vi "Auto Range(SR830).vi"(8 "error in (no error)":errorcluster, 11 "簇":T1={"initialize"=enum."SR830", "6221"={"6221 Resource"="GPIB0::24::INSTR", "Delta status"=FALSE, "电流|RMS(A)"=0.0}, "SR830+6221"={"source"=0, "Current(A)"=0.0, "阻抗(Ohm)"=0.0, "SR830 1"=FALSE, "SR830 2"=FALSE, "SR830 3"=FALSE, "SR830 4"=FALSE, "VISA 1"="", "VISA 2"="", "VISA 3"="", "VISA 4"="", "Reserve 1"=-1, "Reserve 2"=-1, "Reserve 3"=-1, "Reserve 4"=-1, "Sensitivity 1"=-1, "Sensitivity 2"=-1, "Sensitivity 3"=-1, "Sensitivity 4"=-1, "量程入 1"=0, "量程入 2"=0, "量程入 3"=0, "量程入 4"=0}, "2400"={"2400"=FALSE, "VISA"="GPIB0::9::INSTR", "Output Level (0)"=1e-05, "Compliance  Level (0.1)"=10.0}, "ch"={"ch"=[], "current"=[], "change?"=[], "holding current\nwhen change ch?"=FALSE}, "Instrument"={"325 Resource "="GPIB0::13::INSTR", "Input (0:A) 325"=0, "Heater Output (1:1) 325"=1, "340 Resource"="GPIB0::14::INSTR", "Input (0:A) 340"=0, "Loop (0: 1)"=0, "Input (0:B) 340"=1, "Loop (1: 1)"=0, "340 Status"=refnum, "Instrument Type"=enum."PPMS-Rotate", "quantum design"=refnum, "semaphore 325"=refnum, "TCP master instance"=refnum, "M24C Resource"="GPIB0::24::INSTR", "4G supply"="GPIB0::24::INSTR", "Temp Status 24C"=refnum, "Temp"=refnum, "9T信号"=refnum, "limit"={"Field limit"=0.0, "Field rate limit"=0.0, "Temp limit"=0.0, "Temp low limit"=0.0, "Temp rate limit "=0.0}, "4g supply status"=refnum, "vi路径"="", "in-plane"="", "out-plane"="", "in-plane signal"=FALSE, "out-plane signal"=FALSE, "in plane 信号"=refnum, "pzt volt"=refnum, "Aborting"=refnum, "数据文件"=refnum, "warning"=refnum, "750 visa"="", "750 rotate"="", "335 Status 2"=refnum, "335 Resource "="GPIB0::24::INSTR", "Input (0:A) 335"=0, "Input (0:B) 335"=1, "Heater Output (1:1) 335"=1, "semaphore 340"=refnum, "semaphore 335"=refnum, "325 Status"=refnum, "semaphore 750"=refnum, "750 field status"=refnum, "camg 振荡状态"=refnum, "列表框"=refnum, "编辑列表框？"=refnum, "camg Rate"=refnum, "行数"=refnum}, "2614B"={"2614B chA"=FALSE, "2614B chB"=FALSE, "VISA"=""}, "33522b"={"33522b resource name"="GPIB0::16::INSTR", "零电压"=0.0, "最大电压"=148.0, "间隔"=4.0, "最小电压"=-48.0, "PZT Scan?"=FALSE}, "gating type"=enum."2614(daul)", "层数"=0, "行数"=0, "是否处理"=[]} {"Instrument"."Loop (1: 1)" items=["1"=1, "2"=2]; "Instrument"."Loop (0: 1)" items=["1"=1, "2"=2]; "Instrument"."Input (0:B) 340" items=["A", "B", "C", "D"]; "Instrument"."Heater Output (1:1) 335" items=["1"=1, "2"=2]; "Instrument"."Input (0:B) 335" items=["A", "B"]; "Instrument"."Input (0:A) 335" items=["A", "B"]; "Instrument"."Heater Output (1:1) 325" items=["1"=1, "2"=2]; "Instrument"."Input (0:A) 325" items=["A", "B"]; "Instrument"."Input (0:A) 340" items=["1"=1, "2"=2]; "SR830+6221"."Sensitivity 4" items=["Auto Gain"=-1, "2 nV/fA"=0, "5 nV/fA"=1, "10 nV/fA"=2, "20 nV/fA"=3, "50 nV/fA"=4, "100 nV/fA"=5, "200 nV/fA"=6, "500 nV/fA"=7, "1 uV/pA"=8, "2 uV/pA"=9, "5 uV/pA"=10, "10 uV/pA"=11, "20 uV/pA"=12, "50 uV/pA"=13, "100 uV/pA"=14, "200 uV/pA"=15, "500 uV/pA"=16, "1 mV/nA"=17, "2 mV/nA"=18, "5 mV/nA"=19, "10 mV/nA"=20, "20 mV/nA"=21, "50 mV/nA"=22, "100 mV/nA"=23, "200 mV/nA"=24, "500 mV/mA"=25, "1 V/uA"=26]; "SR830+6221"."Sensitivity 3" items=["Auto Gain"=-1, "2 nV/fA"=0, "5 nV/fA"=1, "10 nV/fA"=2, "20 nV/fA"=3, "50 nV/fA"=4, "100 nV/fA"=5, "200 nV/fA"=6, "500 nV/fA"=7, "1 uV/pA"=8, "2 uV/pA"=9, "5 uV/pA"=10, "10 uV/pA"=11, "20 uV/pA"=12, "50 uV/pA"=13, "100 uV/pA"=14, "200 uV/pA"=15, "500 uV/pA"=16, "1 mV/nA"=17, "2 mV/nA"=18, "5 mV/nA"=19, "10 mV/nA"=20, "20 mV/nA"=21, "50 mV/nA"=22, "100 mV/nA"=23, "200 mV/nA"=24, "500 mV/mA"=25, "1 V/uA"=26]; "SR830+6221"."Sensitivity 1" items=["Auto Gain"=-1, "2 nV/fA"=0, "5 nV/fA"=1, "10 nV/fA"=2, "20 nV/fA"=3, "50 nV/fA"=4, "100 nV/fA"=5, "200 nV/fA"=6, "500 nV/fA"=7, "1 uV/pA"=8, "2 uV/pA"=9, "5 uV/pA"=10, "10 uV/pA"=11, "20 uV/pA"=12, "50 uV/pA"=13, "100 uV/pA"=14, "200 uV/pA"=15, "500 uV/pA"=16, "1 mV/nA"=17, "2 mV/nA"=18, "5 mV/nA"=19, "10 mV/nA"=20, "20 mV/nA"=21, "50 mV/nA"=22, "100 mV/nA"=23, "200 mV/nA"=24, "500 mV/mA"=25, "1 V/uA"=26]; "SR830+6221"."Sensitivity 2" items=["Auto Gain"=-1, "2 nV/fA"=0, "5 nV/fA"=1, "10 nV/fA"=2, "20 nV/fA"=3, "50 nV/fA"=4, "100 nV/fA"=5, "200 nV/fA"=6, "500 nV/fA"=7, "1 uV/pA"=8, "2 uV/pA"=9, "5 uV/pA"=10, "10 uV/pA"=11, "20 uV/pA"=12, "50 uV/pA"=13, "100 uV/pA"=14, "200 uV/pA"=15, "500 uV/pA"=16, "1 mV/nA"=17, "2 mV/nA"=18, "5 mV/nA"=19, "10 mV/nA"=20, "20 mV/nA"=21, "50 mV/nA"=22, "100 mV/nA"=23, "200 mV/nA"=24, "500 mV/mA"=25, "1 V/uA"=26]; "SR830+6221"."Reserve 4" items=["Auto Reserve"=-1, "High Reserve"=0, "Normal"=1, "Low Noise"=2]; "SR830+6221"."Reserve 3" items=["Auto Reserve"=-1, "High Reserve"=0, "Normal"=1, "Low Noise"=2]; "SR830+6221"."Reserve 2" items=["Auto Reserve"=-1, "High Reserve"=0, "Normal"=1, "Low Noise"=2]; "SR830+6221"."Reserve 1" items=["Auto Reserve"=-1, "High Reserve"=0, "Normal"=1, "Low Noise"=2]; "SR830+6221"."source" items=["SR830 1", "SR830 2", "SR830 3", "SR830 4"]}) -> (0 "错误输出":errorcluster)   [LabVIEW 2019, in "User lib.lvlib"]
uses:
  ctl/config.ctl
  <vilib>/NI/Modbus Library/API/Master/Modbus Master.lvclass
  ctl/initialize.ctl
  ctl/Instrument.ctl
  ctl/335 state.ctl
  ctl/Instrument Type.ctl
  lib/QDInstrument.dll
  ctl/limit.ctl
  ctl/9T mag field stauts.ctl
  ctl/warning.ctl
  ctl/Gating type.ctl
  User lib.lvlib
  lib/Stanford Research 830/Stanford Research 830.lvlib
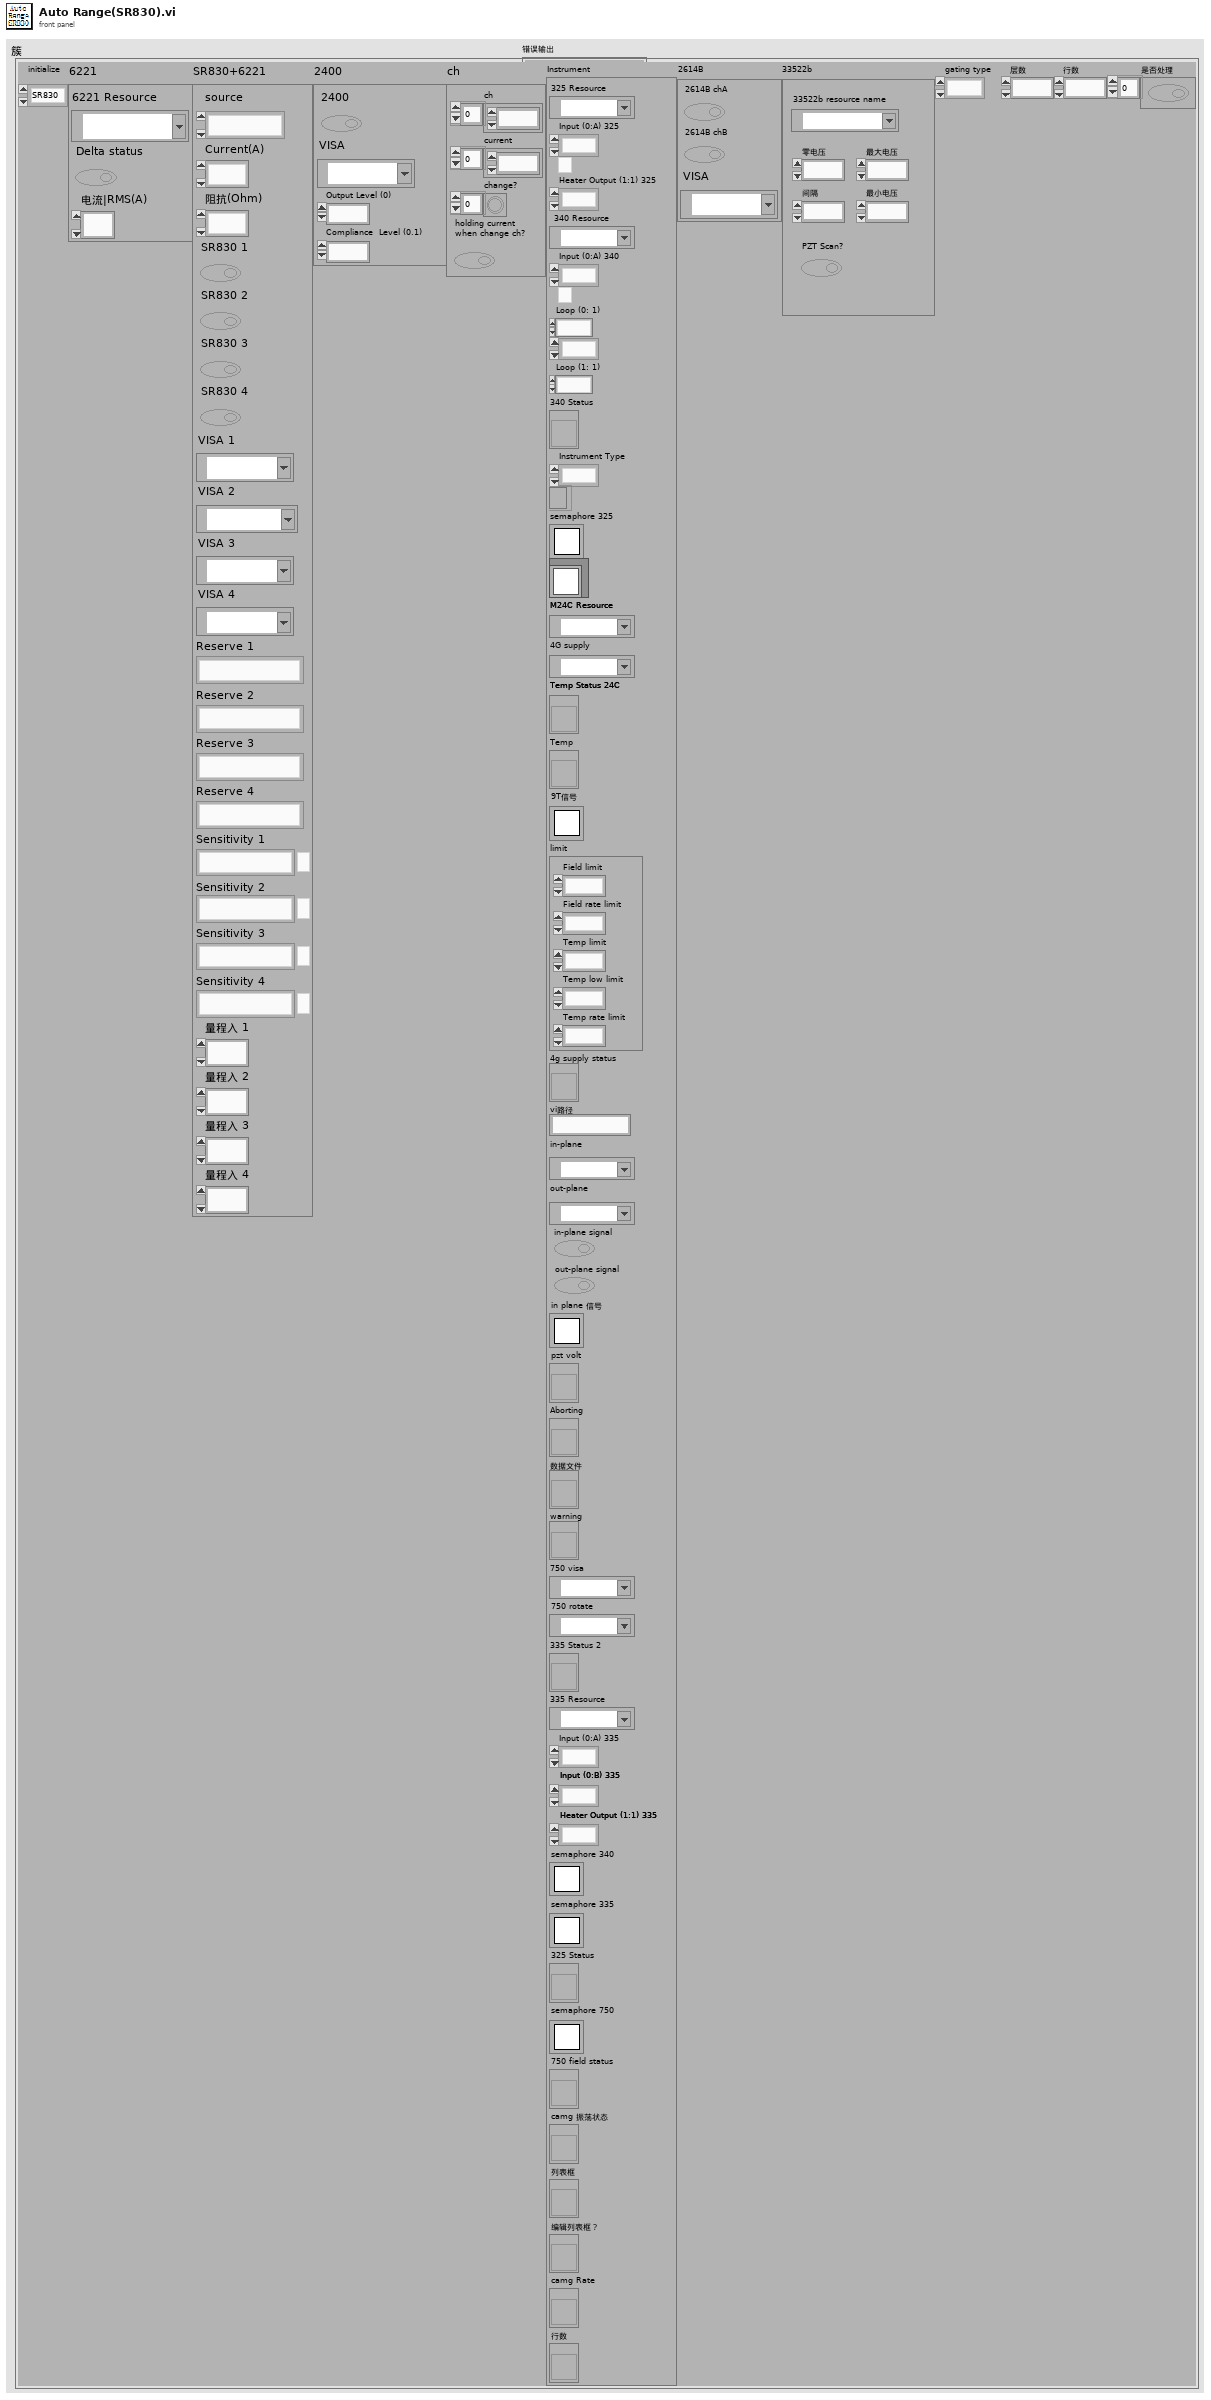
[diagram p1: front panel]
types:
  T1 = typedef "config.ctl" = cluster{"initialize":T2, "6221":cluster{"6221 Resource":refnum<visa-resource-name>, "Delta status":bool, "电流|RMS(A)":dbl}, "SR830+6221":cluster{"source":u16, "Current(A)":dbl, "阻抗(Ohm)":dbl, "SR830 1":bool, "SR830 2":bool, "SR830 3":bool, "SR830 4":bool, "VISA 1":refnum<visa-resource-name>, "VISA 2":refnum<visa-resource-name>, "VISA 3":refnum<visa-resource-name>, "VISA 4":refnum<visa-resource-name>, "Reserve 1":i16, "Reserve 2":i16, "Reserve 3":i16, "Reserve 4":i16, "Sensitivity 1":i16, "Sensitivity 2":i16, "Sensitivity 3":i16, "Sensitivity 4":i16, "量程入 1":i32, "量程入 2":i32, "量程入 3":i32, "量程入 4":i32}, "2400":cluster{"2400":bool, "VISA":refnum<visa-resource-name>, "Output Level (0)":dbl, "Compliance  Level (0.1)":dbl}, "ch":cluster{"ch":i32[], "current":dbl[], "change?":bool[], "holding current\nwhen change ch?":bool}, "Instrument":T3, "2614B":cluster{"2614B chA":bool, "2614B chB":bool, "VISA":refnum<visa-resource-name>}, "33522b":cluster{"33522b resource name":refnum<visa-resource-name>, "零电压":dbl, "最大电压":dbl, "间隔":dbl, "最小电压":dbl, "PZT Scan?":bool}, "gating type":T7, "层数":i32, "行数":i32, "是否处理":bool[]}
  T2 = typedef "initialize.ctl" = enum16{"SR830", "keithley6221-SR830", "Delta", "Delta-tunnelling", "keithley6221-2182-DC", "PZT", "4200"}
  T3 = typedef "Instrument.ctl" = cluster{"325 Resource ":refnum<visa-resource-name>, "Input (0:A) 325":u16, "Heater Output (1:1) 325":u16, "340 Resource":refnum<visa-resource-name>, "Input (0:A) 340":u16, "Loop (0: 1)":u16, "Input (0:B) 340":u16, "Loop (1: 1)":u16, "340 Status":refnum<vi>, "Instrument Type":T4, "quantum design":refnum<k24>, "semaphore 325":T5, "TCP master instance":refnum<class "Modbus Master.lvclass">, "M24C Resource":refnum<visa-resource-name>, "4G supply":refnum<visa-resource-name>, "Temp Status 24C":refnum<vi>, "Temp":refnum<vi>, "9T信号":T5, "limit":T6, "4g supply status":refnum<vi>, "vi路径":string, "in-plane":refnum<visa-resource-name>, "out-plane":refnum<visa-resource-name>, "in-plane signal":bool, "out-plane signal":bool, "in plane 信号":T5, "pzt volt":refnum<vi>, "Aborting":refnum<vi>, "数据文件":refnum<vi>, "warning":refnum<vi>, "750 visa":refnum<visa-resource-name>, "750 rotate":refnum<visa-resource-name>, "335 Status 2":refnum<vi>, "335 Resource ":refnum<visa-resource-name>, "Input (0:A) 335":u16, "Input (0:B) 335":u16, "Heater Output (1:1) 335":u16, "semaphore 340":T5, "semaphore 335":T5, "325 Status":refnum<vi>, "semaphore 750":T5, "750 field status":refnum<vi>, "camg 振荡状态":refnum<vi>, "列表框":refnum<vi>, "编辑列表框？":refnum<vi>, "camg Rate":refnum<vi>, "行数":refnum<vi>}
  T4 = typedef "Instrument Type.ctl" = enum16{"PPMS", "VersaLab", "DynaCool", "SVSM", "PPMS-Rotate", "Lakeshore335", "lengtou2", "9T mag", "9T cmag rotate", "test"}
  T5 = typedef "Semaphore RefNum" = refnum<k1>
  T6 = typedef "limit.ctl" = cluster{"Field limit":dbl, "Field rate limit":dbl, "Temp limit":dbl, "Temp low limit":dbl, "Temp rate limit ":dbl}
  T7 = typedef "Gating type.ctl" = enum32{"null", "2614(daul)", "2400", "6517B"}
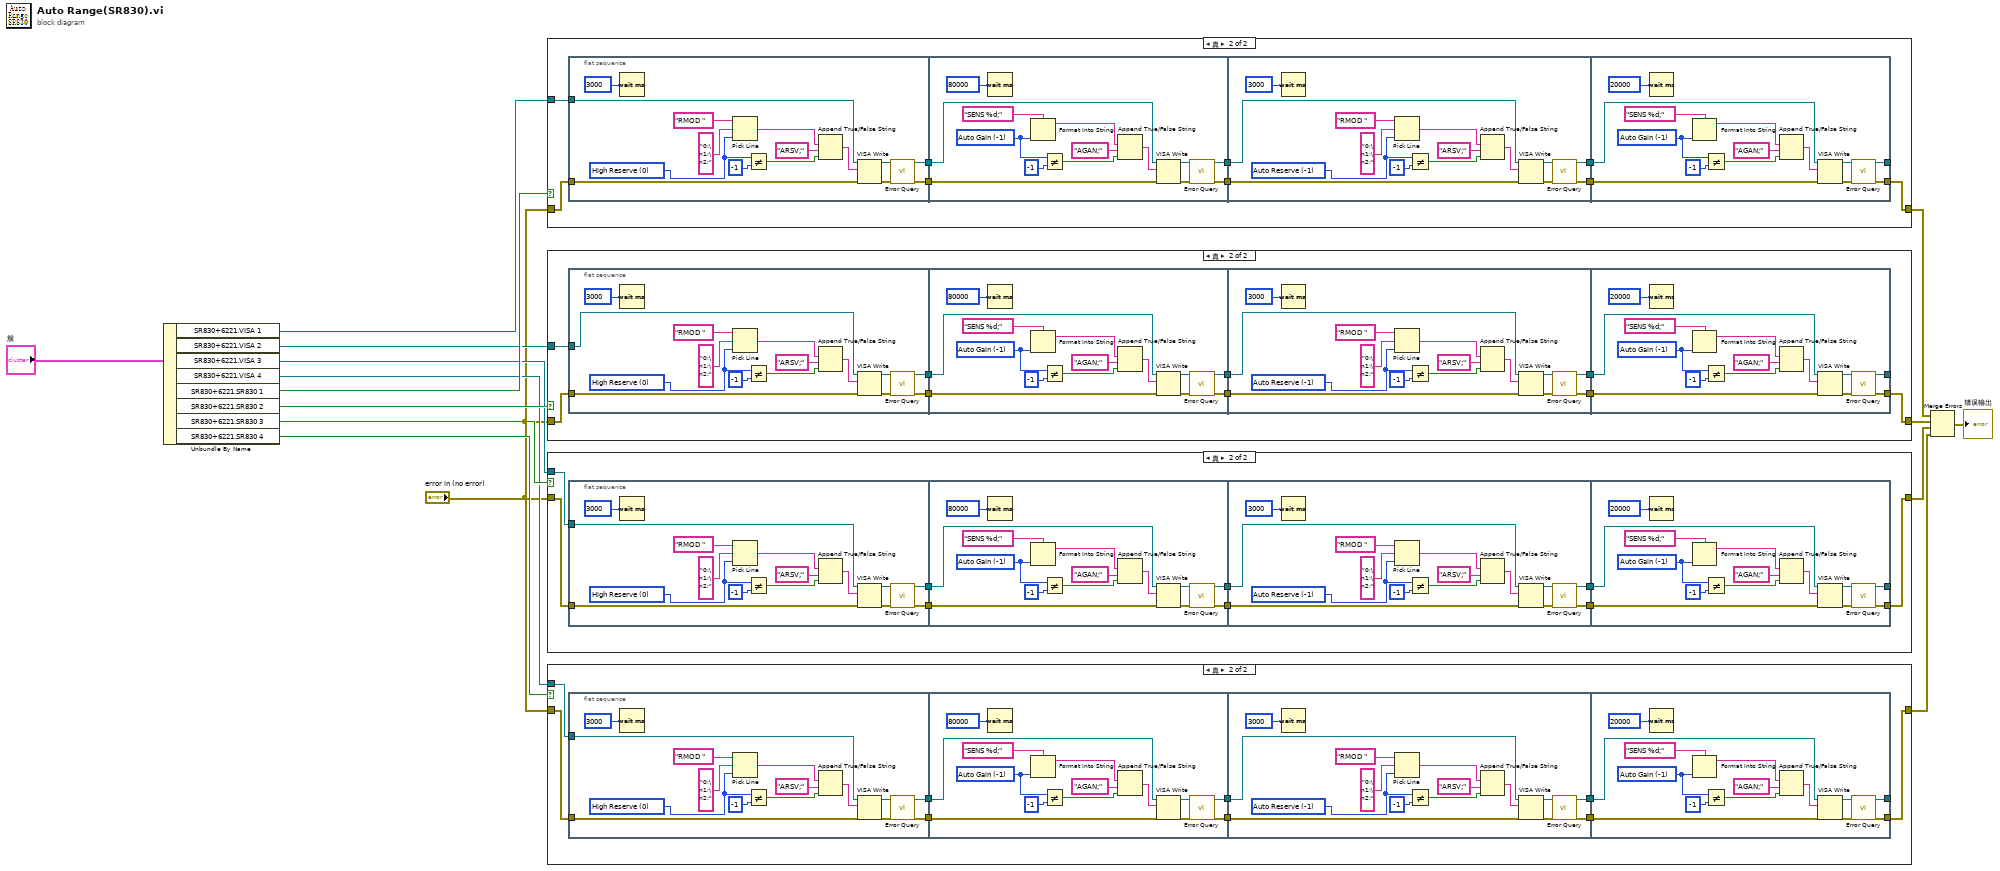
[diagram p0: block diagram]
diagram:
  n1 = Unbundle By Name("簇") -> ("SR830+6221.VISA 1"=w9:refnum<visa-resource-name>, "SR830+6221.VISA 2"=w7:refnum<visa-resource-name>, "SR830+6221.VISA 3"=w5:refnum<visa-resource-name>, "SR830+6221.VISA 4"=w3:refnum<visa-resource-name>, "SR830+6221.SR830 1"=w13:bool, "SR830+6221.SR830 2"=w12:bool, "SR830+6221.SR830 3"=w11:bool, "SR830+6221.SR830 4"=w10:bool)
  n2 = case shown="真" w13 {
    tunnel: w9 -> [_ w19]
    tunnel: "error in (no error)" -> [w16 w18]
    tunnel: [w16 w17] -> w8
    frame False {
    }
    frame True {
      n3 = flat-sequence {
        tunnel: w19 -> [w31]
        tunnel: w18 -> [w30]
        tunnel: [w27] -> w25
        tunnel: [w28] -> w24
        tunnel: [w43] -> w23
        tunnel: [w42] -> w22
        tunnel: w25 -> [w45]
        tunnel: w24 -> [w44]
        tunnel: w23 -> [w60]
        tunnel: w22 -> [w61]
        tunnel: [w57] -> w20
        tunnel: [w56] -> w21
        tunnel: w21 -> [w73]
        tunnel: w20 -> [w74]
        tunnel: [w71] -> w17
        tunnel: [w70] -> _
        frame #0 {
          w38 = i16 0 items=["Auto Reserve"=-1, "High Reserve"=0, "Normal"=1, "Low Noise"=2] ("Dynamic Reserve (-1: Auto Reserve)")
          n4 = Wait (ms)(milliseconds to wait=u32 3000 ("等待时间（毫秒）")) -> ()  [unwired: 1 out]
          n5 = Pick Line(string ("")="RMOD ", multi-line string="0;\n1;\n2;", line index=w38) -> (output string=w40:string)
          n6 = Not Equal?(x=w38, y=i16 -1) -> (x != y?=w39:bool)
          n7 = Append True/False String(1:w39, 2:"ARSV;" ("false string"), 3:w40) -> (0:w29:string)  [unwired: 1 in]
          n8 = VISA Write(VISA resource name=w31, write buffer=w29, error in (no error)=w30) -> (VISA resource name out=w32:refnum<visa-resource-name>, error out=w33:errorcluster)  [unwired: 1 out]
          n9 = call "Error Query.vi"("error in (no error)"=w33, "VISA resource name"=w32) -> ("error out"=w27:errorcluster, "VISA resource name out"=w28:refnum<visa-resource-name>)  [unwired: 7 in, 1 out]
        }
        frame #1 {
          w48 = i16 -1 items=["Auto Gain"=-1, "2 nV/fA"=0, "5 nV/fA"=1, "10 nV/fA"=2, "20 nV/fA"=3, "50 nV/fA"=4, "100 nV/fA"=5, "200 nV/fA"=6, "500 nV/fA"=7, "1 uV/pA"=8, "2 uV/pA"=9, "5 uV/pA"=10, "10 uV/pA"=11, "20 uV/pA"=12, "50 uV/pA"=13, "100 uV/pA"=14, "200 uV/pA"=15, "500 uV/pA"=16, "1 mV/nA"=17, "2 mV/nA"=18, "5 mV/nA"=19, "10 mV/nA"=20, "20 mV/nA"=21, "50 mV/nA"=22, "100 mV/nA"=23, "200 mV/nA"=24, "500 mV/mA"=25, "1 V/uA"=26] ("Sensitivity (-1: Auto gain)")
          n10 = Wait (ms)(milliseconds to wait=u32 80000 ("等待时间（毫秒）")) -> ()  [unwired: 1 out]
          n11 = Format Into String(format string="SENS %d;", w48) -> (resulting string=w51:string)  [unwired: 2 in, 1 out]
          n12 = Not Equal?(x=w48, y=i16 -1) -> (x != y?=w50:bool)
          n13 = Append True/False String(1:w50, 2:"AGAN;" ("false string"), 3:w51) -> (0:w54:string)  [unwired: 1 in]
          n14 = VISA Write(VISA resource name=w44, write buffer=w54, error in (no error)=w45) -> (VISA resource name out=w52:refnum<visa-resource-name>, error out=w53:errorcluster)  [unwired: 1 out]
          n15 = call "Error Query.vi"("error in (no error)"=w53, "VISA resource name"=w52) -> ("error out"=w43:errorcluster, "VISA resource name out"=w42:refnum<visa-resource-name>)  [unwired: 7 in, 1 out]
        }
        frame #2 {
          w67 = i16 -1 items=["Auto Reserve"=-1, "High Reserve"=0, "Normal"=1, "Low Noise"=2] ("Dynamic Reserve (-1: Auto Reserve)")
          n16 = Wait (ms)(milliseconds to wait=u32 3000 ("等待时间（毫秒）")) -> ()  [unwired: 1 out]
          n17 = Pick Line(string ("")="RMOD ", multi-line string="0;\n1;\n2;", line index=w67) -> (output string=w69:string)
          n18 = Not Equal?(x=w67, y=i16 -1) -> (x != y?=w68:bool)
          n19 = Append True/False String(1:w68, 2:"ARSV;" ("false string"), 3:w69) -> (0:w62:string)  [unwired: 1 in]
          n20 = VISA Write(VISA resource name=w61, write buffer=w62, error in (no error)=w60) -> (VISA resource name out=w58:refnum<visa-resource-name>, error out=w59:errorcluster)  [unwired: 1 out]
          n21 = call "Error Query.vi"("error in (no error)"=w59, "VISA resource name"=w58) -> ("error out"=w56:errorcluster, "VISA resource name out"=w57:refnum<visa-resource-name>)  [unwired: 7 in, 1 out]
        }
        frame #3 {
          w77 = i16 -1 items=["Auto Gain"=-1, "2 nV/fA"=0, "5 nV/fA"=1, "10 nV/fA"=2, "20 nV/fA"=3, "50 nV/fA"=4, "100 nV/fA"=5, "200 nV/fA"=6, "500 nV/fA"=7, "1 uV/pA"=8, "2 uV/pA"=9, "5 uV/pA"=10, "10 uV/pA"=11, "20 uV/pA"=12, "50 uV/pA"=13, "100 uV/pA"=14, "200 uV/pA"=15, "500 uV/pA"=16, "1 mV/nA"=17, "2 mV/nA"=18, "5 mV/nA"=19, "10 mV/nA"=20, "20 mV/nA"=21, "50 mV/nA"=22, "100 mV/nA"=23, "200 mV/nA"=24, "500 mV/mA"=25, "1 V/uA"=26] ("Sensitivity (-1: Auto gain)")
          n22 = Wait (ms)(milliseconds to wait=u32 20000 ("等待时间（毫秒）")) -> ()  [unwired: 1 out]
          n23 = Format Into String(format string="SENS %d;", w77) -> (resulting string=w80:string)  [unwired: 2 in, 1 out]
          n24 = Not Equal?(x=w77, y=i16 -1) -> (x != y?=w79:bool)
          n25 = Append True/False String(1:w79, 2:"AGAN;" ("false string"), 3:w80) -> (0:w83:string)  [unwired: 1 in]
          n26 = VISA Write(VISA resource name=w74, write buffer=w83, error in (no error)=w73) -> (VISA resource name out=w81:refnum<visa-resource-name>, error out=w82:errorcluster)  [unwired: 1 out]
          n27 = call "Error Query.vi"("error in (no error)"=w82, "VISA resource name"=w81) -> ("error out"=w71:errorcluster, "VISA resource name out"=w70:refnum<visa-resource-name>)  [unwired: 7 in, 1 out]
        }
      }
    }
  }
  n28 = case shown="真" w12 {
    tunnel: w7 -> [_ w87]
    tunnel: "error in (no error)" -> [w84 w86]
    tunnel: [w84 w85] -> w6
    frame False {
    }
    frame True {
      n29 = flat-sequence {
        tunnel: w87 -> [w99]
        tunnel: w86 -> [w98]
        tunnel: [w95] -> w93
        tunnel: [w96] -> w92
        tunnel: [w111] -> w91
        tunnel: [w110] -> w90
        tunnel: w93 -> [w113]
        tunnel: w92 -> [w112]
        tunnel: w91 -> [w128]
        tunnel: w90 -> [w129]
        tunnel: [w125] -> w88
        tunnel: [w124] -> w89
        tunnel: w89 -> [w141]
        tunnel: w88 -> [w142]
        tunnel: [w139] -> w85
        tunnel: [w138] -> _
        frame #0 {
          w106 = i16 0 items=["Auto Reserve"=-1, "High Reserve"=0, "Normal"=1, "Low Noise"=2] ("Dynamic Reserve (-1: Auto Reserve)")
          n30 = Wait (ms)(milliseconds to wait=u32 3000 ("等待时间（毫秒）")) -> ()  [unwired: 1 out]
          n31 = Pick Line(string ("")="RMOD ", multi-line string="0;\n1;\n2;", line index=w106) -> (output string=w108:string)
          n32 = Not Equal?(x=w106, y=i16 -1) -> (x != y?=w107:bool)
          n33 = Append True/False String(1:w107, 2:"ARSV;" ("false string"), 3:w108) -> (0:w97:string)  [unwired: 1 in]
          n34 = VISA Write(VISA resource name=w99, write buffer=w97, error in (no error)=w98) -> (VISA resource name out=w100:refnum<visa-resource-name>, error out=w101:errorcluster)  [unwired: 1 out]
          n35 = call "Error Query.vi"("error in (no error)"=w101, "VISA resource name"=w100) -> ("error out"=w95:errorcluster, "VISA resource name out"=w96:refnum<visa-resource-name>)  [unwired: 7 in, 1 out]
        }
        frame #1 {
          w116 = i16 -1 items=["Auto Gain"=-1, "2 nV/fA"=0, "5 nV/fA"=1, "10 nV/fA"=2, "20 nV/fA"=3, "50 nV/fA"=4, "100 nV/fA"=5, "200 nV/fA"=6, "500 nV/fA"=7, "1 uV/pA"=8, "2 uV/pA"=9, "5 uV/pA"=10, "10 uV/pA"=11, "20 uV/pA"=12, "50 uV/pA"=13, "100 uV/pA"=14, "200 uV/pA"=15, "500 uV/pA"=16, "1 mV/nA"=17, "2 mV/nA"=18, "5 mV/nA"=19, "10 mV/nA"=20, "20 mV/nA"=21, "50 mV/nA"=22, "100 mV/nA"=23, "200 mV/nA"=24, "500 mV/mA"=25, "1 V/uA"=26] ("Sensitivity (-1: Auto gain)")
          n36 = Wait (ms)(milliseconds to wait=u32 80000 ("等待时间（毫秒）")) -> ()  [unwired: 1 out]
          n37 = Format Into String(format string="SENS %d;", w116) -> (resulting string=w119:string)  [unwired: 2 in, 1 out]
          n38 = Not Equal?(x=w116, y=i16 -1) -> (x != y?=w118:bool)
          n39 = Append True/False String(1:w118, 2:"AGAN;" ("false string"), 3:w119) -> (0:w122:string)  [unwired: 1 in]
          n40 = VISA Write(VISA resource name=w112, write buffer=w122, error in (no error)=w113) -> (VISA resource name out=w120:refnum<visa-resource-name>, error out=w121:errorcluster)  [unwired: 1 out]
          n41 = call "Error Query.vi"("error in (no error)"=w121, "VISA resource name"=w120) -> ("error out"=w111:errorcluster, "VISA resource name out"=w110:refnum<visa-resource-name>)  [unwired: 7 in, 1 out]
        }
        frame #2 {
          w135 = i16 -1 items=["Auto Reserve"=-1, "High Reserve"=0, "Normal"=1, "Low Noise"=2] ("Dynamic Reserve (-1: Auto Reserve)")
          n42 = Wait (ms)(milliseconds to wait=u32 3000 ("等待时间（毫秒）")) -> ()  [unwired: 1 out]
          n43 = Pick Line(string ("")="RMOD ", multi-line string="0;\n1;\n2;", line index=w135) -> (output string=w137:string)
          n44 = Not Equal?(x=w135, y=i16 -1) -> (x != y?=w136:bool)
          n45 = Append True/False String(1:w136, 2:"ARSV;" ("false string"), 3:w137) -> (0:w130:string)  [unwired: 1 in]
          n46 = VISA Write(VISA resource name=w129, write buffer=w130, error in (no error)=w128) -> (VISA resource name out=w126:refnum<visa-resource-name>, error out=w127:errorcluster)  [unwired: 1 out]
          n47 = call "Error Query.vi"("error in (no error)"=w127, "VISA resource name"=w126) -> ("error out"=w124:errorcluster, "VISA resource name out"=w125:refnum<visa-resource-name>)  [unwired: 7 in, 1 out]
        }
        frame #3 {
          w145 = i16 -1 items=["Auto Gain"=-1, "2 nV/fA"=0, "5 nV/fA"=1, "10 nV/fA"=2, "20 nV/fA"=3, "50 nV/fA"=4, "100 nV/fA"=5, "200 nV/fA"=6, "500 nV/fA"=7, "1 uV/pA"=8, "2 uV/pA"=9, "5 uV/pA"=10, "10 uV/pA"=11, "20 uV/pA"=12, "50 uV/pA"=13, "100 uV/pA"=14, "200 uV/pA"=15, "500 uV/pA"=16, "1 mV/nA"=17, "2 mV/nA"=18, "5 mV/nA"=19, "10 mV/nA"=20, "20 mV/nA"=21, "50 mV/nA"=22, "100 mV/nA"=23, "200 mV/nA"=24, "500 mV/mA"=25, "1 V/uA"=26] ("Sensitivity (-1: Auto gain)")
          n48 = Wait (ms)(milliseconds to wait=u32 20000 ("等待时间（毫秒）")) -> ()  [unwired: 1 out]
          n49 = Format Into String(format string="SENS %d;", w145) -> (resulting string=w148:string)  [unwired: 2 in, 1 out]
          n50 = Not Equal?(x=w145, y=i16 -1) -> (x != y?=w147:bool)
          n51 = Append True/False String(1:w147, 2:"AGAN;" ("false string"), 3:w148) -> (0:w151:string)  [unwired: 1 in]
          n52 = VISA Write(VISA resource name=w142, write buffer=w151, error in (no error)=w141) -> (VISA resource name out=w149:refnum<visa-resource-name>, error out=w150:errorcluster)  [unwired: 1 out]
          n53 = call "Error Query.vi"("error in (no error)"=w150, "VISA resource name"=w149) -> ("error out"=w139:errorcluster, "VISA resource name out"=w138:refnum<visa-resource-name>)  [unwired: 7 in, 1 out]
        }
      }
    }
  }
  n54 = case shown="真" w11 {
    tunnel: w5 -> [_ w155]
    tunnel: "error in (no error)" -> [w152 w154]
    tunnel: [w152 w153] -> w4
    frame False {
    }
    frame True {
      n55 = flat-sequence {
        tunnel: w155 -> [w167]
        tunnel: w154 -> [w166]
        tunnel: [w163] -> w161
        tunnel: [w164] -> w160
        tunnel: [w179] -> w159
        tunnel: [w178] -> w158
        tunnel: w161 -> [w181]
        tunnel: w160 -> [w180]
        tunnel: w159 -> [w196]
        tunnel: w158 -> [w197]
        tunnel: [w193] -> w156
        tunnel: [w192] -> w157
        tunnel: w157 -> [w209]
        tunnel: w156 -> [w210]
        tunnel: [w207] -> w153
        tunnel: [w206] -> _
        frame #0 {
          w174 = i16 0 items=["Auto Reserve"=-1, "High Reserve"=0, "Normal"=1, "Low Noise"=2] ("Dynamic Reserve (-1: Auto Reserve)")
          n56 = Wait (ms)(milliseconds to wait=u32 3000 ("等待时间（毫秒）")) -> ()  [unwired: 1 out]
          n57 = Pick Line(string ("")="RMOD ", multi-line string="0;\n1;\n2;", line index=w174) -> (output string=w176:string)
          n58 = Not Equal?(x=w174, y=i16 -1) -> (x != y?=w175:bool)
          n59 = Append True/False String(1:w175, 2:"ARSV;" ("false string"), 3:w176) -> (0:w165:string)  [unwired: 1 in]
          n60 = VISA Write(VISA resource name=w167, write buffer=w165, error in (no error)=w166) -> (VISA resource name out=w168:refnum<visa-resource-name>, error out=w169:errorcluster)  [unwired: 1 out]
          n61 = call "Error Query.vi"("error in (no error)"=w169, "VISA resource name"=w168) -> ("error out"=w163:errorcluster, "VISA resource name out"=w164:refnum<visa-resource-name>)  [unwired: 7 in, 1 out]
        }
        frame #1 {
          w184 = i16 -1 items=["Auto Gain"=-1, "2 nV/fA"=0, "5 nV/fA"=1, "10 nV/fA"=2, "20 nV/fA"=3, "50 nV/fA"=4, "100 nV/fA"=5, "200 nV/fA"=6, "500 nV/fA"=7, "1 uV/pA"=8, "2 uV/pA"=9, "5 uV/pA"=10, "10 uV/pA"=11, "20 uV/pA"=12, "50 uV/pA"=13, "100 uV/pA"=14, "200 uV/pA"=15, "500 uV/pA"=16, "1 mV/nA"=17, "2 mV/nA"=18, "5 mV/nA"=19, "10 mV/nA"=20, "20 mV/nA"=21, "50 mV/nA"=22, "100 mV/nA"=23, "200 mV/nA"=24, "500 mV/mA"=25, "1 V/uA"=26] ("Sensitivity (-1: Auto gain)")
          n62 = Wait (ms)(milliseconds to wait=u32 80000 ("等待时间（毫秒）")) -> ()  [unwired: 1 out]
          n63 = Format Into String(format string="SENS %d;", w184) -> (resulting string=w187:string)  [unwired: 2 in, 1 out]
          n64 = Not Equal?(x=w184, y=i16 -1) -> (x != y?=w186:bool)
          n65 = Append True/False String(1:w186, 2:"AGAN;" ("false string"), 3:w187) -> (0:w190:string)  [unwired: 1 in]
          n66 = VISA Write(VISA resource name=w180, write buffer=w190, error in (no error)=w181) -> (VISA resource name out=w188:refnum<visa-resource-name>, error out=w189:errorcluster)  [unwired: 1 out]
          n67 = call "Error Query.vi"("error in (no error)"=w189, "VISA resource name"=w188) -> ("error out"=w179:errorcluster, "VISA resource name out"=w178:refnum<visa-resource-name>)  [unwired: 7 in, 1 out]
        }
        frame #2 {
          w203 = i16 -1 items=["Auto Reserve"=-1, "High Reserve"=0, "Normal"=1, "Low Noise"=2] ("Dynamic Reserve (-1: Auto Reserve)")
          n68 = Wait (ms)(milliseconds to wait=u32 3000 ("等待时间（毫秒）")) -> ()  [unwired: 1 out]
          n69 = Pick Line(string ("")="RMOD ", multi-line string="0;\n1;\n2;", line index=w203) -> (output string=w205:string)
          n70 = Not Equal?(x=w203, y=i16 -1) -> (x != y?=w204:bool)
          n71 = Append True/False String(1:w204, 2:"ARSV;" ("false string"), 3:w205) -> (0:w198:string)  [unwired: 1 in]
          n72 = VISA Write(VISA resource name=w197, write buffer=w198, error in (no error)=w196) -> (VISA resource name out=w194:refnum<visa-resource-name>, error out=w195:errorcluster)  [unwired: 1 out]
          n73 = call "Error Query.vi"("error in (no error)"=w195, "VISA resource name"=w194) -> ("error out"=w192:errorcluster, "VISA resource name out"=w193:refnum<visa-resource-name>)  [unwired: 7 in, 1 out]
        }
        frame #3 {
          w213 = i16 -1 items=["Auto Gain"=-1, "2 nV/fA"=0, "5 nV/fA"=1, "10 nV/fA"=2, "20 nV/fA"=3, "50 nV/fA"=4, "100 nV/fA"=5, "200 nV/fA"=6, "500 nV/fA"=7, "1 uV/pA"=8, "2 uV/pA"=9, "5 uV/pA"=10, "10 uV/pA"=11, "20 uV/pA"=12, "50 uV/pA"=13, "100 uV/pA"=14, "200 uV/pA"=15, "500 uV/pA"=16, "1 mV/nA"=17, "2 mV/nA"=18, "5 mV/nA"=19, "10 mV/nA"=20, "20 mV/nA"=21, "50 mV/nA"=22, "100 mV/nA"=23, "200 mV/nA"=24, "500 mV/mA"=25, "1 V/uA"=26] ("Sensitivity (-1: Auto gain)")
          n74 = Wait (ms)(milliseconds to wait=u32 20000 ("等待时间（毫秒）")) -> ()  [unwired: 1 out]
          n75 = Format Into String(format string="SENS %d;", w213) -> (resulting string=w216:string)  [unwired: 2 in, 1 out]
          n76 = Not Equal?(x=w213, y=i16 -1) -> (x != y?=w215:bool)
          n77 = Append True/False String(1:w215, 2:"AGAN;" ("false string"), 3:w216) -> (0:w219:string)  [unwired: 1 in]
          n78 = VISA Write(VISA resource name=w210, write buffer=w219, error in (no error)=w209) -> (VISA resource name out=w217:refnum<visa-resource-name>, error out=w218:errorcluster)  [unwired: 1 out]
          n79 = call "Error Query.vi"("error in (no error)"=w218, "VISA resource name"=w217) -> ("error out"=w207:errorcluster, "VISA resource name out"=w206:refnum<visa-resource-name>)  [unwired: 7 in, 1 out]
        }
      }
    }
  }
  n80 = case shown="真" w10 {
    tunnel: w3 -> [_ w223]
    tunnel: "error in (no error)" -> [w220 w222]
    tunnel: [w220 w221] -> w1
    frame False {
    }
    frame True {
      n81 = flat-sequence {
        tunnel: w223 -> [w235]
        tunnel: w222 -> [w234]
        tunnel: [w231] -> w229
        tunnel: [w232] -> w228
        tunnel: [w247] -> w227
        tunnel: [w246] -> w226
        tunnel: w229 -> [w249]
        tunnel: w228 -> [w248]
        tunnel: w227 -> [w264]
        tunnel: w226 -> [w265]
        tunnel: [w261] -> w224
        tunnel: [w260] -> w225
        tunnel: w225 -> [w277]
        tunnel: w224 -> [w278]
        tunnel: [w275] -> w221
        tunnel: [w274] -> _
        frame #0 {
          w242 = i16 0 items=["Auto Reserve"=-1, "High Reserve"=0, "Normal"=1, "Low Noise"=2] ("Dynamic Reserve (-1: Auto Reserve)")
          n82 = Wait (ms)(milliseconds to wait=u32 3000 ("等待时间（毫秒）")) -> ()  [unwired: 1 out]
          n83 = Pick Line(string ("")="RMOD ", multi-line string="0;\n1;\n2;", line index=w242) -> (output string=w244:string)
          n84 = Not Equal?(x=w242, y=i16 -1) -> (x != y?=w243:bool)
          n85 = Append True/False String(1:w243, 2:"ARSV;" ("false string"), 3:w244) -> (0:w233:string)  [unwired: 1 in]
          n86 = VISA Write(VISA resource name=w235, write buffer=w233, error in (no error)=w234) -> (VISA resource name out=w236:refnum<visa-resource-name>, error out=w237:errorcluster)  [unwired: 1 out]
          n87 = call "Error Query.vi"("error in (no error)"=w237, "VISA resource name"=w236) -> ("error out"=w231:errorcluster, "VISA resource name out"=w232:refnum<visa-resource-name>)  [unwired: 7 in, 1 out]
        }
        frame #1 {
          w252 = i16 -1 items=["Auto Gain"=-1, "2 nV/fA"=0, "5 nV/fA"=1, "10 nV/fA"=2, "20 nV/fA"=3, "50 nV/fA"=4, "100 nV/fA"=5, "200 nV/fA"=6, "500 nV/fA"=7, "1 uV/pA"=8, "2 uV/pA"=9, "5 uV/pA"=10, "10 uV/pA"=11, "20 uV/pA"=12, "50 uV/pA"=13, "100 uV/pA"=14, "200 uV/pA"=15, "500 uV/pA"=16, "1 mV/nA"=17, "2 mV/nA"=18, "5 mV/nA"=19, "10 mV/nA"=20, "20 mV/nA"=21, "50 mV/nA"=22, "100 mV/nA"=23, "200 mV/nA"=24, "500 mV/mA"=25, "1 V/uA"=26] ("Sensitivity (-1: Auto gain)")
          n88 = Wait (ms)(milliseconds to wait=u32 80000 ("等待时间（毫秒）")) -> ()  [unwired: 1 out]
          n89 = Format Into String(format string="SENS %d;", w252) -> (resulting string=w255:string)  [unwired: 2 in, 1 out]
          n90 = Not Equal?(x=w252, y=i16 -1) -> (x != y?=w254:bool)
          n91 = Append True/False String(1:w254, 2:"AGAN;" ("false string"), 3:w255) -> (0:w258:string)  [unwired: 1 in]
          n92 = VISA Write(VISA resource name=w248, write buffer=w258, error in (no error)=w249) -> (VISA resource name out=w256:refnum<visa-resource-name>, error out=w257:errorcluster)  [unwired: 1 out]
          n93 = call "Error Query.vi"("error in (no error)"=w257, "VISA resource name"=w256) -> ("error out"=w247:errorcluster, "VISA resource name out"=w246:refnum<visa-resource-name>)  [unwired: 7 in, 1 out]
        }
        frame #2 {
          w271 = i16 -1 items=["Auto Reserve"=-1, "High Reserve"=0, "Normal"=1, "Low Noise"=2] ("Dynamic Reserve (-1: Auto Reserve)")
          n94 = Wait (ms)(milliseconds to wait=u32 3000 ("等待时间（毫秒）")) -> ()  [unwired: 1 out]
          n95 = Pick Line(string ("")="RMOD ", multi-line string="0;\n1;\n2;", line index=w271) -> (output string=w273:string)
          n96 = Not Equal?(x=w271, y=i16 -1) -> (x != y?=w272:bool)
          n97 = Append True/False String(1:w272, 2:"ARSV;" ("false string"), 3:w273) -> (0:w266:string)  [unwired: 1 in]
          n98 = VISA Write(VISA resource name=w265, write buffer=w266, error in (no error)=w264) -> (VISA resource name out=w262:refnum<visa-resource-name>, error out=w263:errorcluster)  [unwired: 1 out]
          n99 = call "Error Query.vi"("error in (no error)"=w263, "VISA resource name"=w262) -> ("error out"=w260:errorcluster, "VISA resource name out"=w261:refnum<visa-resource-name>)  [unwired: 7 in, 1 out]
        }
        frame #3 {
          w281 = i16 -1 items=["Auto Gain"=-1, "2 nV/fA"=0, "5 nV/fA"=1, "10 nV/fA"=2, "20 nV/fA"=3, "50 nV/fA"=4, "100 nV/fA"=5, "200 nV/fA"=6, "500 nV/fA"=7, "1 uV/pA"=8, "2 uV/pA"=9, "5 uV/pA"=10, "10 uV/pA"=11, "20 uV/pA"=12, "50 uV/pA"=13, "100 uV/pA"=14, "200 uV/pA"=15, "500 uV/pA"=16, "1 mV/nA"=17, "2 mV/nA"=18, "5 mV/nA"=19, "10 mV/nA"=20, "20 mV/nA"=21, "50 mV/nA"=22, "100 mV/nA"=23, "200 mV/nA"=24, "500 mV/mA"=25, "1 V/uA"=26] ("Sensitivity (-1: Auto gain)")
          n100 = Wait (ms)(milliseconds to wait=u32 20000 ("等待时间（毫秒）")) -> ()  [unwired: 1 out]
          n101 = Format Into String(format string="SENS %d;", w281) -> (resulting string=w284:string)  [unwired: 2 in, 1 out]
          n102 = Not Equal?(x=w281, y=i16 -1) -> (x != y?=w283:bool)
          n103 = Append True/False String(1:w283, 2:"AGAN;" ("false string"), 3:w284) -> (0:w287:string)  [unwired: 1 in]
          n104 = VISA Write(VISA resource name=w278, write buffer=w287, error in (no error)=w277) -> (VISA resource name out=w285:refnum<visa-resource-name>, error out=w286:errorcluster)  [unwired: 1 out]
          n105 = call "Error Query.vi"("error in (no error)"=w286, "VISA resource name"=w285) -> ("error out"=w275:errorcluster, "VISA resource name out"=w274:refnum<visa-resource-name>)  [unwired: 7 in, 1 out]
        }
      }
    }
  }
  n106 = Merge Errors(w8, w6, w4, w1) -> (→"错误输出":errorcluster)
